vi "Apply Filters.vi"(8 "error in (no error)":errorcluster, 11 "State in":T1={"Raw File Data"="", "Deduplicated String Array"=[], "1-Entries"=[], "2-Entries"=[], "3-Entries"=[], "Bounds"={"M-Min"=0, "M-Max"=1023, "S-Min"=0, "S-Max"=1023}, "Matched ADC Values - Nearest"=[], "Match Entry Indices - Nearest"=[], "Filtered 1-Entries"=[], "Filtered 2-Entries"=[], "Filtered 3-Entries"=[], "Total Duration"=0.0, "Matched ADC Values - Largest"=[], "Match Entry Indices - Largest"=[]}) -> (0 "error out":errorcluster, 3 "State out":T1={"Raw File Data"="", "Deduplicated String Array"=[], "1-Entries"=[], "2-Entries"=[], "3-Entries"=[], "Bounds"={"M-Min"=0, "M-Max"=1023, "S-Min"=0, "S-Max"=1023}, "Matched ADC Values - Nearest"=[], "Match Entry Indices - Nearest"=[], "Filtered 1-Entries"=[], "Filtered 2-Entries"=[], "Filtered 3-Entries"=[], "Total Duration"=0.0, "Matched ADC Values - Largest"=[], "Match Entry Indices - Largest"=[]})   [LabVIEW 2019, in "Muon Data Post-Processing.lvlib"]
uses:
  Muon Data Post-Processing.lvlib
  State Data.ctl
  File Entry.ctl
  ADC Bounds.ctl
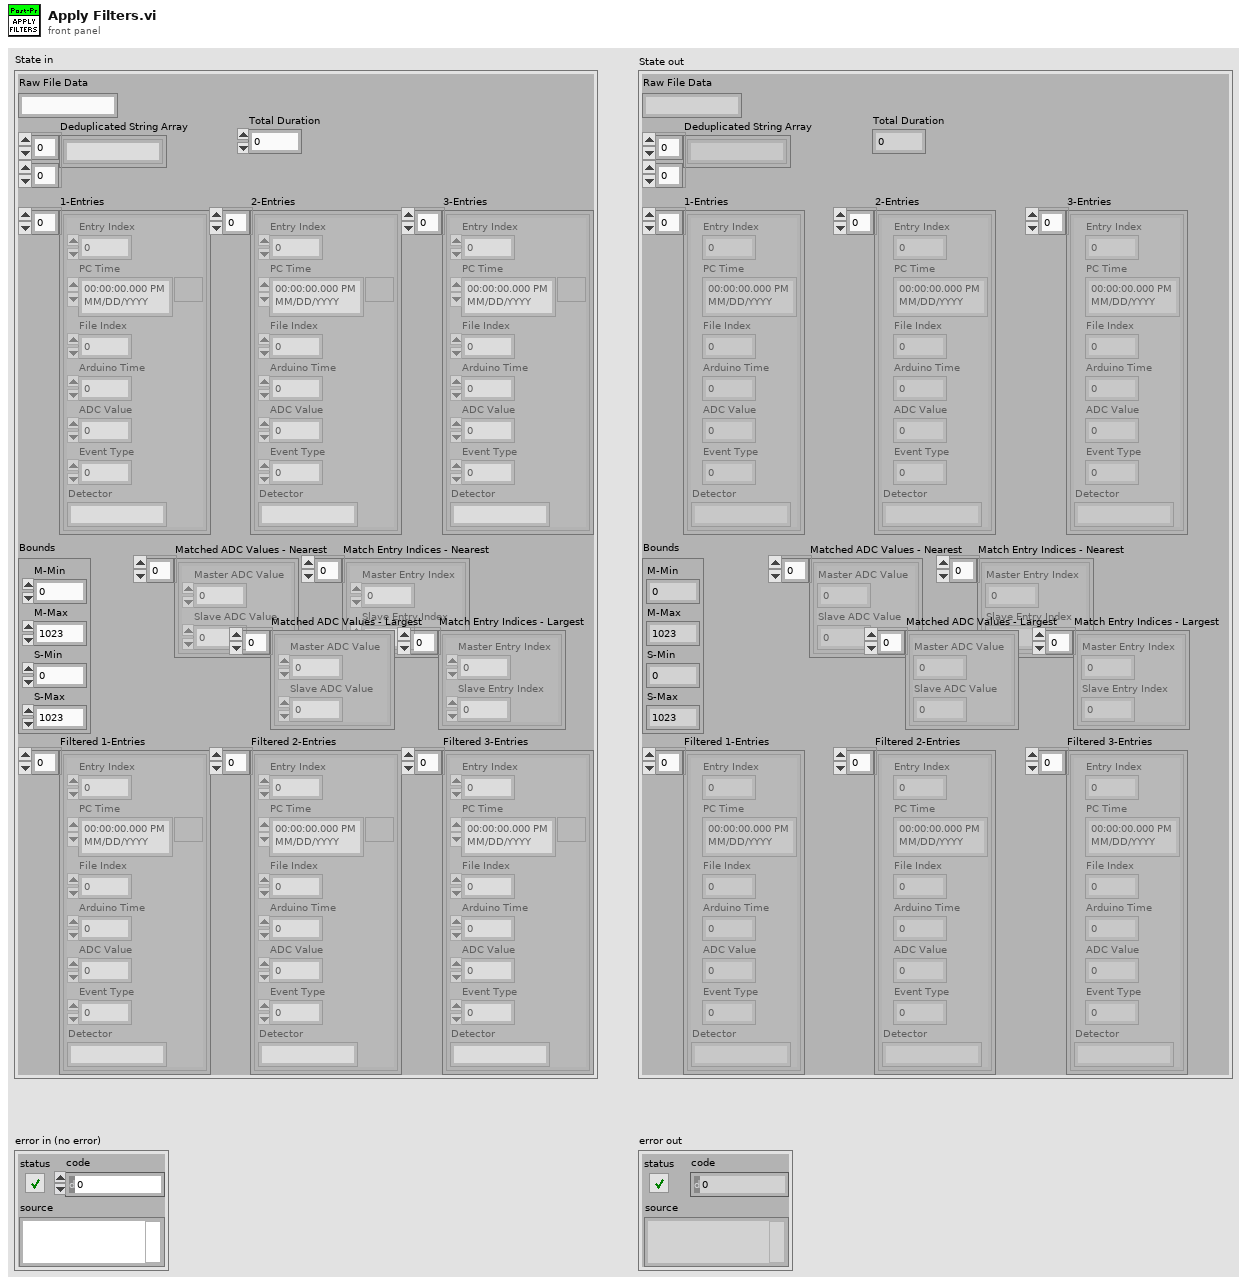
[diagram p1: front panel]
types:
  T1 = typedef "Muon Data Post-Processing.lvlib/State Data.ctl" = cluster{"Raw File Data":string, "Deduplicated String Array":string[][], "1-Entries":T2[], "2-Entries":T2[], "3-Entries":T2[], "Bounds":T3, "Matched ADC Values - Nearest":cluster{"Master ADC Value":i32, "Slave ADC Value":i32}[], "Match Entry Indices - Nearest":cluster{"Master Entry Index":i32, "Slave Entry Index":i32}[], "Filtered 1-Entries":T2[], "Filtered 2-Entries":T2[], "Filtered 3-Entries":T2[], "Total Duration":dbl, "Matched ADC Values - Largest":cluster{"Master ADC Value":i32, "Slave ADC Value":i32}[], "Match Entry Indices - Largest":cluster{"Master Entry Index":i32, "Slave Entry Index":i32}[]}
  T2 = typedef "Muon Data Post-Processing.lvlib/File Entry.ctl" = cluster{"Entry Index":i32, "PC Time":timestamp, "File Index":i32, "Arduino Time":i32, "ADC Value":i32, "Event Type":i32, "Detector":string}
  T3 = typedef "Muon Data Post-Processing.lvlib/ADC Bounds.ctl" = cluster{"M-Min":u16, "M-Max":u16, "S-Min":u16, "S-Max":u16}
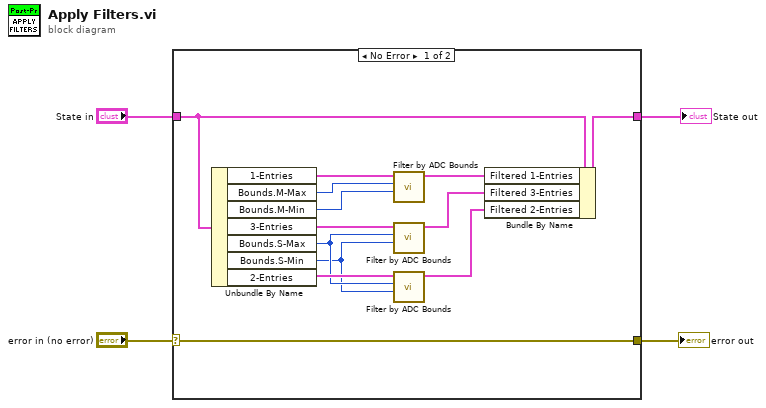
[diagram p0: block diagram]
diagram:
  n1 = case shown="No Error" "error in (no error)" {
    selector: "error in (no error)" -> [w17 w18]
    tunnel: [w8 w19] -> w3
    tunnel: "State in" -> [w9 w19]
    tunnel: [w17 w18] -> w1
    frame No Error {
      n2 = Unbundle By Name(w9) -> ("1-Entries"=w16:T2[], "Bounds.M-Max"=w15:u16, "Bounds.M-Min"=w14:u16, "3-Entries"=w13:T2[], "Bounds.S-Max"=w11:u16, "Bounds.S-Min"=w10:u16, "2-Entries"=w12:T2[])
      n3 = call "Filter by ADC Bounds.vi"("Min"=w14, "Max"=w15, "Entries"=w16) -> ("Filtered Entries"=w5:T2[])  [unwired: 7 in, 1 out]
      n4 = call "Filter by ADC Bounds.vi"("Min"=w10, "Max"=w11, "Entries"=w13) -> ("Filtered Entries"=w6:T2[])  [unwired: 7 in, 1 out]
      n5 = call "Filter by ADC Bounds.vi"("Min"=w10, "Max"=w11, "Entries"=w12) -> ("Filtered Entries"=w7:T2[])  [unwired: 7 in, 1 out]
      n6 = Bundle By Name(cluster=w9, "Filtered 1-Entries"=w5, "Filtered 3-Entries"=w6, "Filtered 2-Entries"=w7) -> (w8:T1)
    }
    frame Error {
    }
  }
  "State out" <- w3
  "error out" <- w1
